vi "FaceRecognition_realtime_detection_usingPCA.vi"() -> ()   [LabVIEW 2017]
uses:
  <vilib>/userdefined/High Color/IMAQdx.ctl
  <vilib>/vision/driver/NI_Vision_Acquisition_Software.lvlib
  <vilib>/vision/NI_Vision_Development_Module.lvlib
panel:
  out "添加的数组":i32[](array[numeric])
  out "Faces":T1[](array[typedef]) {"Rotation" format="%.2f"; "Left" scale=0.0..1024.0; "Right" scale=0.0..1024.0}
  in  "error in":errorcluster
  in  "选项卡控件":enum32{"实时监测", "图像检测"}(tab)
  out "匹配到DB中图像":T2(plugin-control)
  in  "识别方法":u16(ring)=1 items=["模板匹配", "KL变换（调用Matlab）"]
  out "识别结果":string
  in  "是否去背景":bool
  out "Segment image":T2(plugin-control)
  out "检测到人脸":bool
  out "识别时间ms":dbl format="%#.2g"
  in  "切换":bool
  out "Live Image":T2(plugin-control)
  in  "选择相机":T3="cam0"
  in  "停止":bool
  out "Image 2":T2(plugin-control)
  out "识别的图像路径":path
  out "取人脸区域":T2(plugin-control)
  out "识别结果（KL变换）":T2(plugin-control)
  out "输入图像识别结果":string
  out "检测出人脸":bool
  out "Process结果":T2(plugin-control)
  out "Selected img":T2(plugin-control)
  in  "选择图像":bool
  in  "切换 2":bool
  in  "停止2":bool
  # "人脸识别系统"
  # "人脸识别系统"
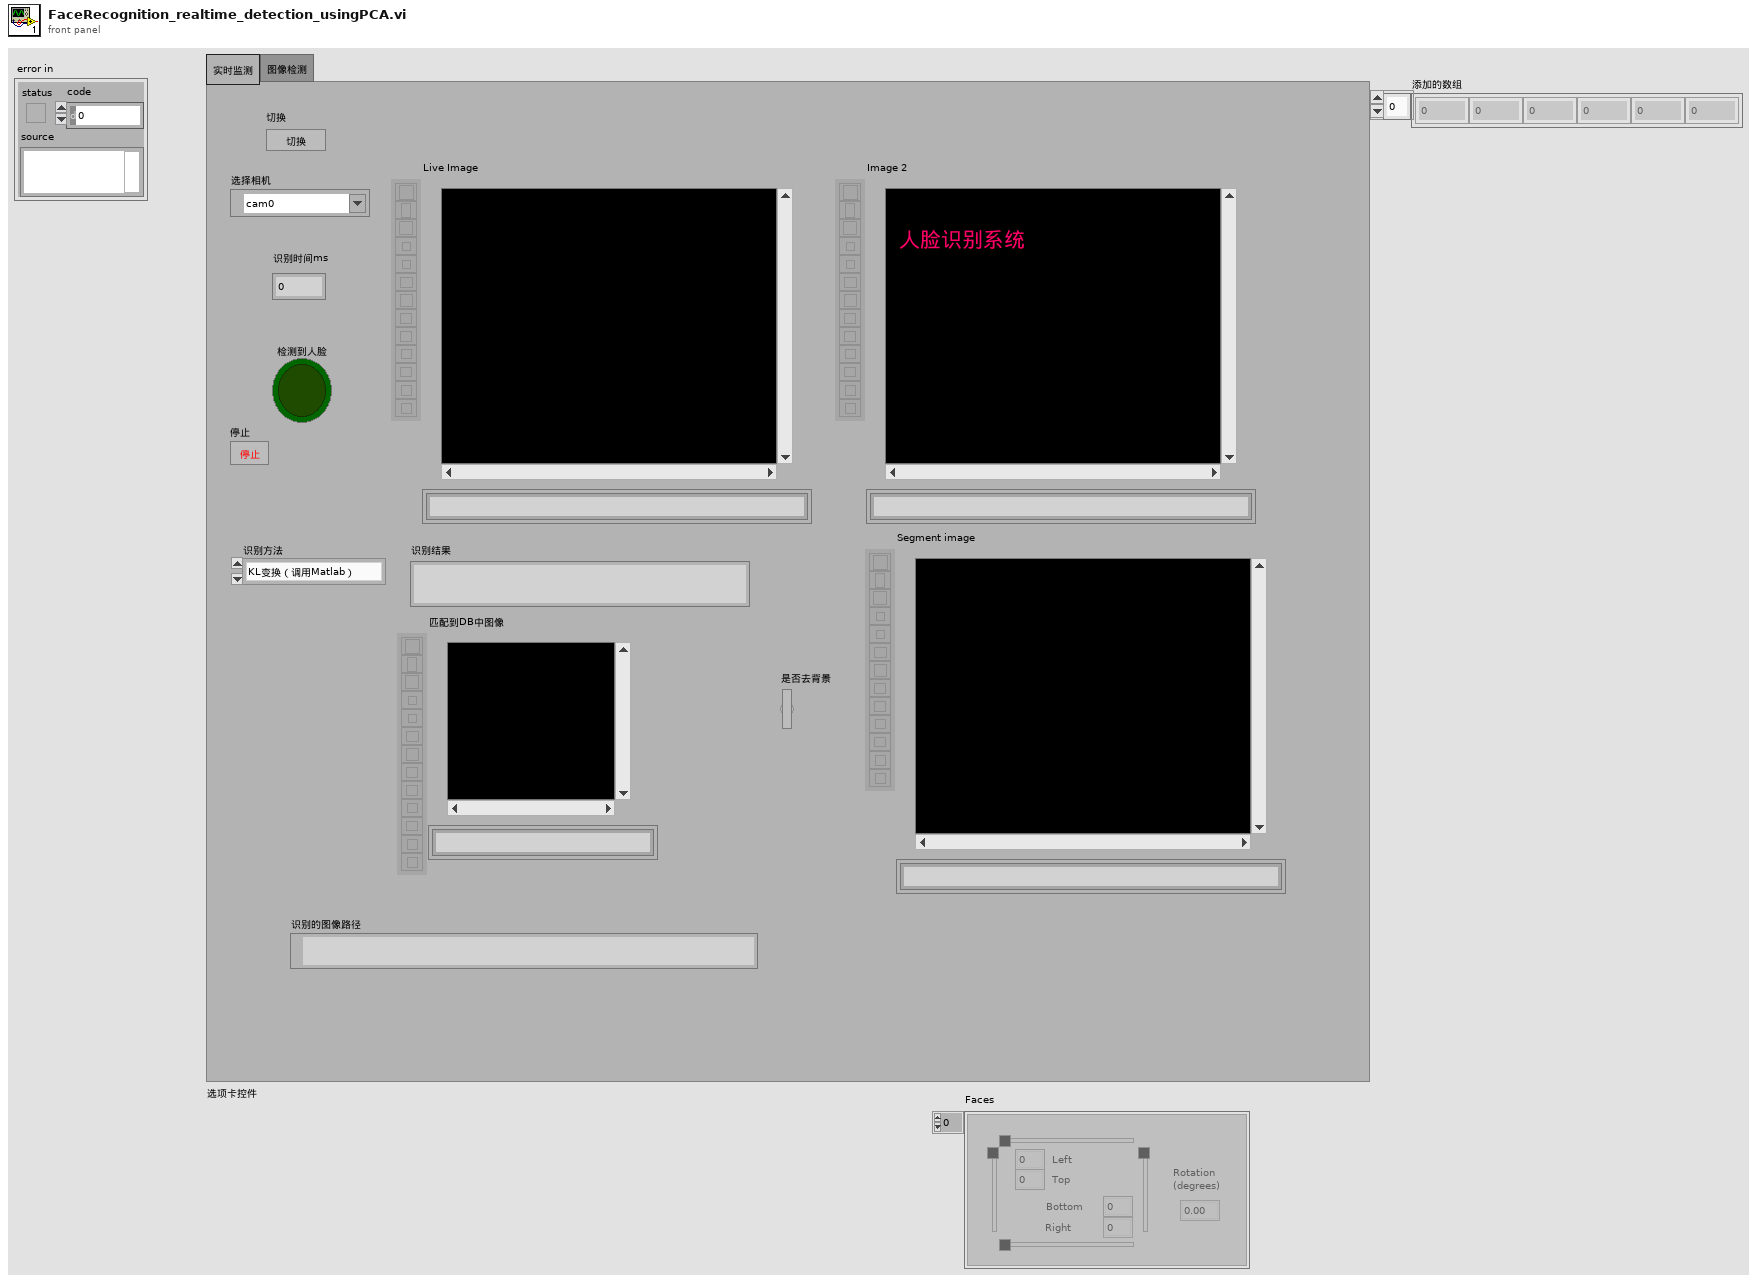
[diagram p1: front panel]
types:
  T1 = typedef "IMAQ Rectangle" = cluster{"Left":i32, "Top":i32, "Right":i32, "Bottom":i32, "Rotation":dbl}
  T2 = typedef "IMAQ Image.ctl" = refnum<image>
  T3 = typedef "IMAQdx.ctl" = refnum<k21>
  T4 = typedef "Image Type" = u32
  T5 = enum32{"Average", "Min", "Max", "Clear  if < ", "Clear  if < or =", "Clear  if =", "Clear  if > or =", "Clear  if >"}
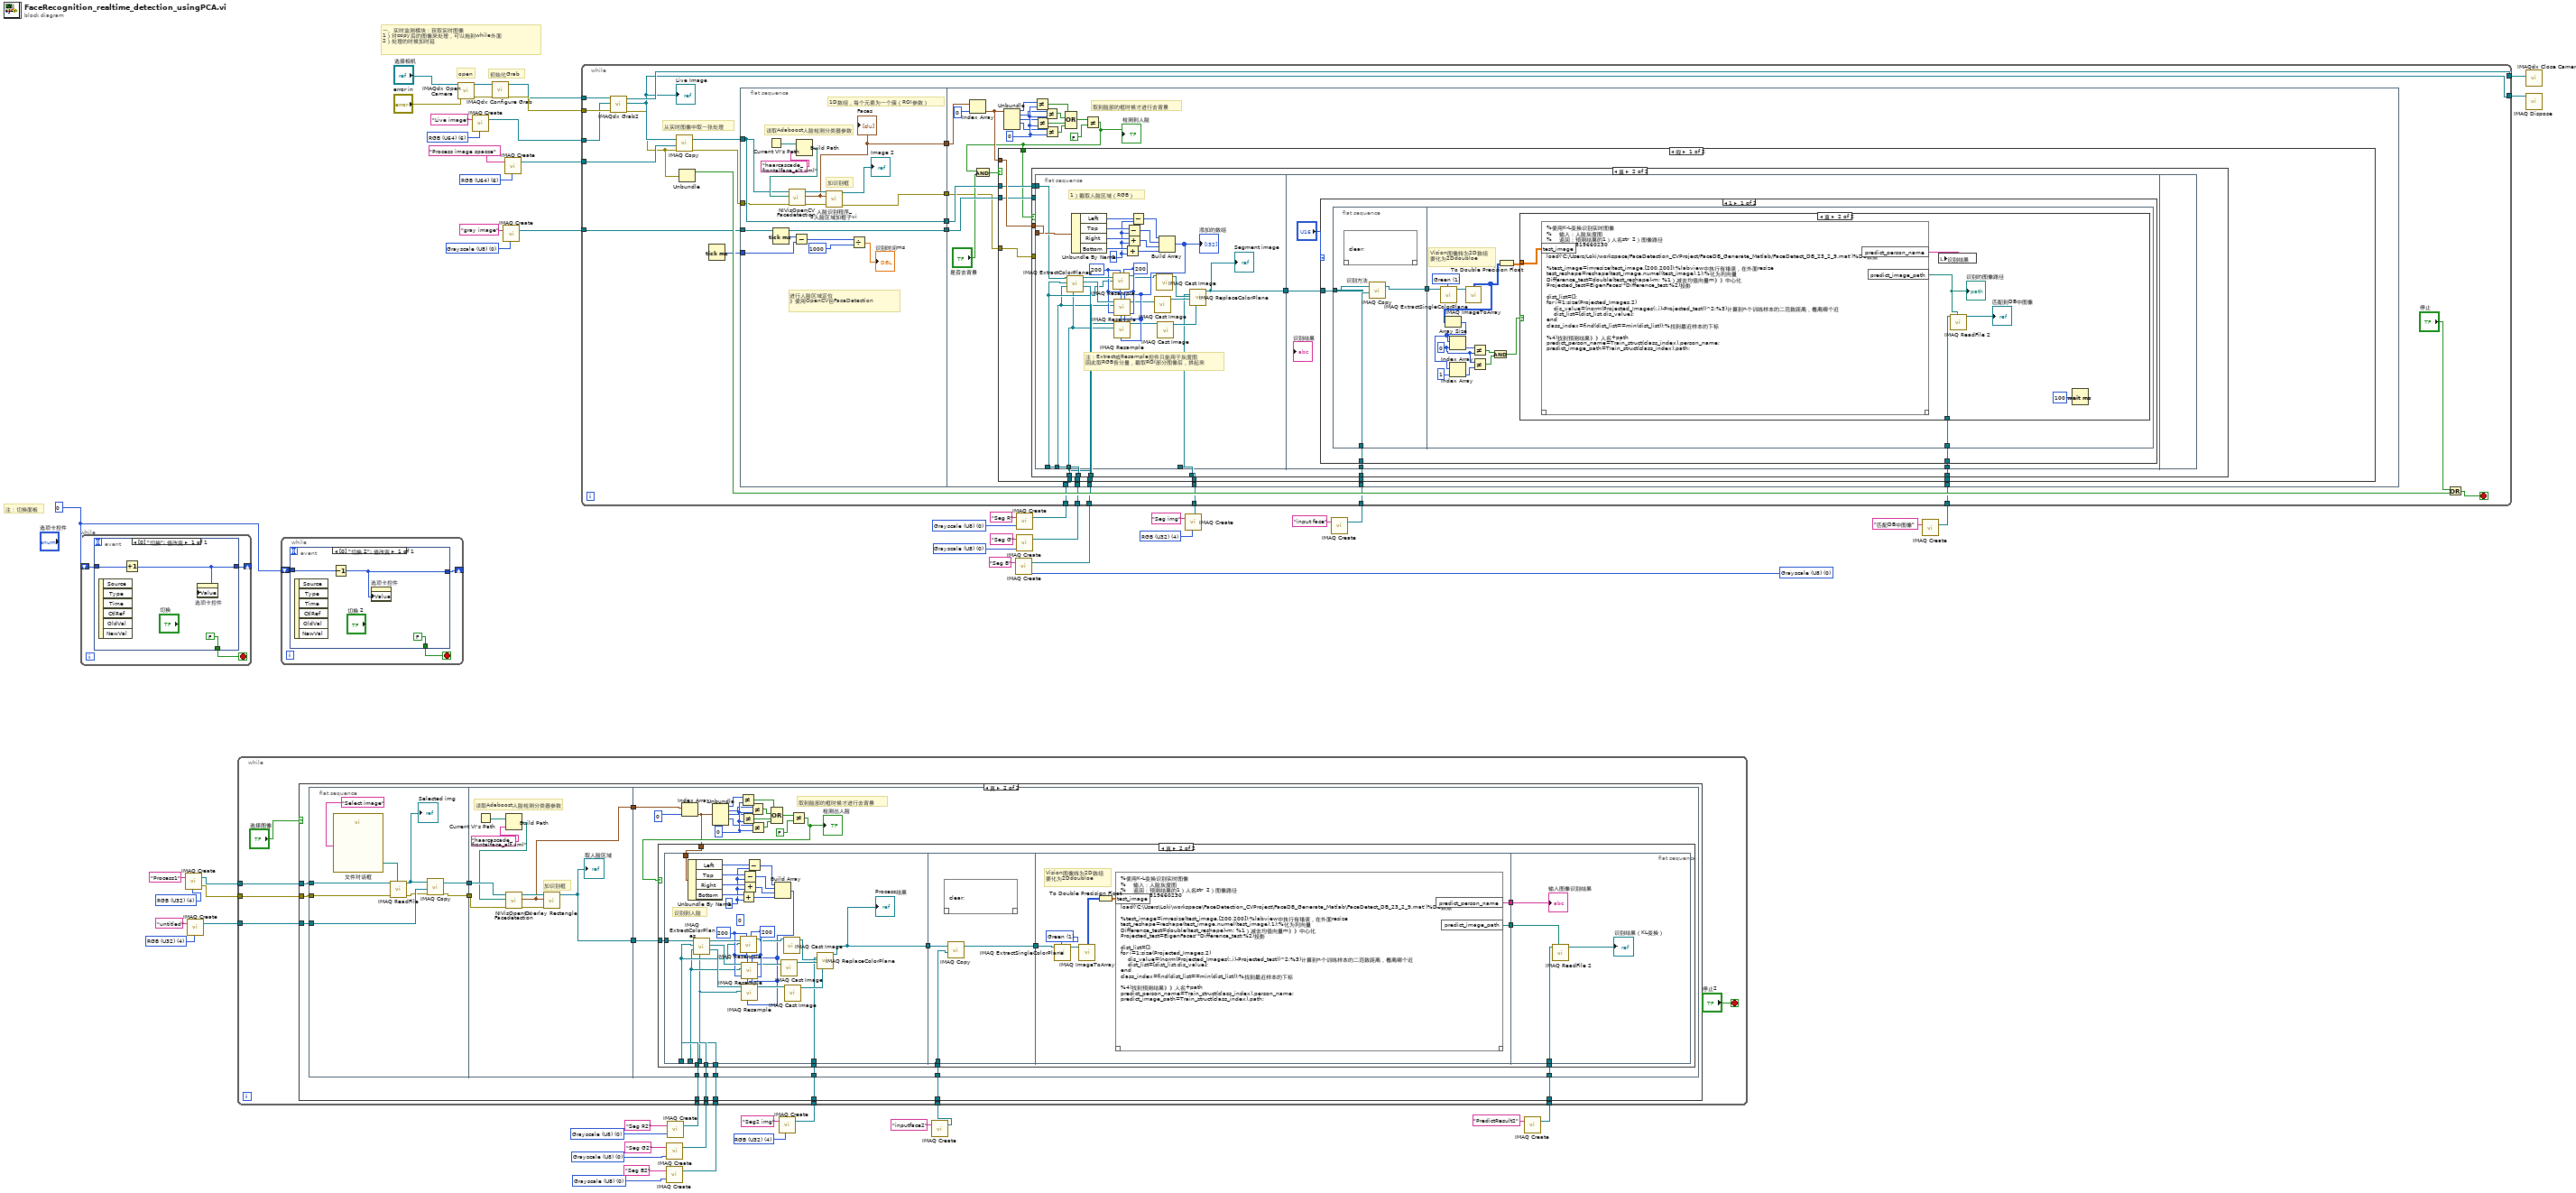
[diagram p0: block diagram]
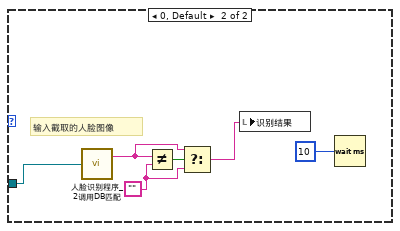
[diagram p6: hidden frame]
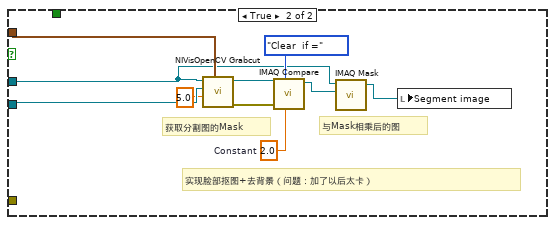
[diagram p7: hidden frame]
diagram:
  w2 = T4 4 items=["Grayscale (U8)", "Grayscale (I16)", "Grayscale (SGL)", "Complex (CSG)", "RGB (U32)", "HSL (U32)", "RGB (U64)", "Grayscale (U16)"] ("Image Type")
  w11 = T4 0 items=["Grayscale (U8)", "Grayscale (I16)", "Grayscale (SGL)", "Complex (CSG)", "RGB (U32)", "HSL (U32)", "RGB (U64)", "Grayscale (U16)"] ("Image Type")
  w12 = T4 0 items=["Grayscale (U8)", "Grayscale (I16)", "Grayscale (SGL)", "Complex (CSG)", "RGB (U32)", "HSL (U32)", "RGB (U64)", "Grayscale (U16)"] ("Image Type")
  w13 = T4 0 items=["Grayscale (U8)", "Grayscale (I16)", "Grayscale (SGL)", "Complex (CSG)", "RGB (U32)", "HSL (U32)", "RGB (U64)", "Grayscale (U16)"] ("Image Type")
  w23 = T4 4 items=["Grayscale (U8)", "Grayscale (I16)", "Grayscale (SGL)", "Complex (CSG)", "RGB (U32)", "HSL (U32)", "RGB (U64)", "Grayscale (U16)"] ("Image Type")
  w28 = T4 0 items=["Grayscale (U8)", "Grayscale (I16)", "Grayscale (SGL)", "Complex (CSG)", "RGB (U32)", "HSL (U32)", "RGB (U64)", "Grayscale (U16)"] ("Image Type")
  w29 = T4 0 items=["Grayscale (U8)", "Grayscale (I16)", "Grayscale (SGL)", "Complex (CSG)", "RGB (U32)", "HSL (U32)", "RGB (U64)", "Grayscale (U16)"] ("Image Type")
  w30 = T4 0 items=["Grayscale (U8)", "Grayscale (I16)", "Grayscale (SGL)", "Complex (CSG)", "RGB (U32)", "HSL (U32)", "RGB (U64)", "Grayscale (U16)"] ("Image Type")
  w35 = T4 0 items=["Grayscale (U8)", "Grayscale (I16)", "Grayscale (SGL)", "Complex (CSG)", "RGB (U32)", "HSL (U32)", "RGB (U64)", "Grayscale (U16)"] ("Image Type")
  w38 = T4 4 items=["Grayscale (U8)", "Grayscale (I16)", "Grayscale (SGL)", "Complex (CSG)", "RGB (U32)", "HSL (U32)", "RGB (U64)", "Grayscale (U16)"] ("Image Type")
  w42 = T4 4 items=["Grayscale (U8)", "Grayscale (I16)", "Grayscale (SGL)", "Complex (CSG)", "RGB (U32)", "HSL (U32)", "RGB (U64)", "Grayscale (U16)"] ("Image Type")
  w44 = 0
  w47 = T4 6 items=["Grayscale (U8)", "Grayscale (I16)", "Grayscale (SGL)", "Complex (CSG)", "RGB (U32)", "HSL (U32)", "RGB (U64)", "Grayscale (U16)"] ("Image Type")
  w45 = T4 6 items=["Grayscale (U8)", "Grayscale (I16)", "Grayscale (SGL)", "Complex (CSG)", "RGB (U32)", "HSL (U32)", "RGB (U64)", "Grayscale (U16)"] ("Image Type")
  # "注：切换面板"
  # "初始化Grab"
  # "open"
  # "一、实时监测模块：获取实时图像\n1）对copy后的图像来处理，可以拖到while外面\n2）处理的时候加时延"
  n1 = while {
    shift-right: [w59] -> _
    shift-left: w44 -> [w60]
    stop <- w58 stop-if-true
    n2 = event shown="[0] \"切换\": 值改变" {
      selector: _ -> [_]
      dyn-events: _ -> [_]
      timeout: _ -> [_]
      tunnel: w60 -> [w63]
      tunnel: [w62] -> w59
      tunnel: [FALSE] -> w58
      event "切换": Value Change {
        n3 = event-data() -> ()  [unwired: 1 in, 6 out]
        n4 = Increment(x=w63) -> (x+1=w62:i32)
        n5 = property on="选项卡控件" class="TabCtl (严格)"("Value"=w62) -> ()  [unwired: 2 in, 2 out]
      }
    }
  }
  n6 = call "IMAQ Create"("Image Name"="Process1", "Image Type"=w42) -> ("New Image"=w41:T2, "error out"=w40:errorcluster)  [unwired: 3 in]
  n7 = call "IMAQ Create"("Image Name"="untitled", "Image Type"=w38) -> ("New Image"=w37:T2)  [unwired: 3 in, 1 out]
  n8 = while {
    shift-right: [w64] -> _
    shift-left: w44 -> [w65]
    stop <- w66 stop-if-true
    n9 = event shown="[0] \"切换 2\": 值改变" {
      selector: _ -> [_]
      dyn-events: _ -> [_]
      timeout: _ -> [_]
      tunnel: [FALSE] -> w66
      tunnel: w65 -> [w68]
      tunnel: [w67] -> w64
      event "切换 2": Value Change {
        n10 = event-data() -> ()  [unwired: 1 in, 6 out]
        n11 = Decrement(x=w68) -> (x-1=w67:i32)
        n12 = property on="选项卡控件" class="TabCtl (严格)"("Value"=w67) -> ()  [unwired: 2 in, 2 out]
      }
    }
  }
  n13 = call <vilib>:"IMAQdx Open Camera.vi"("error in"="error in", "Session In"="选择相机") -> ("error out"=w50:errorcluster, "Session Out"=w49:T3)  [unwired: 8 in]
  n14 = call "IMAQ Create"("Image Name"="Live image", "Image Type"=w45) -> ("New Image"=w54:T2)  [unwired: 3 in, 1 out]
  n15 = call <vilib>:"IMAQdx Configure Grab.vi"("error in"=w50, "Session In"=w49) -> ("error out"=w53:errorcluster, "Session Out"=w52:T3)  [unwired: 8 in]
  n16 = call "IMAQ Create"("Image Name"="gray image", "Image Type"=w35) -> ("New Image"=w34:T2)  [unwired: 3 in, 1 out]
  n17 = call "IMAQ Create"("Image Name"="Process image spacce", "Image Type"=w47) -> ("New Image"=w56:T2)  [unwired: 3 in, 1 out]
  n18 = call "IMAQ Create"("Image Name"="Seg B2", "Image Type"=w11) -> ("New Image"=w8:T2)  [unwired: 3 in, 1 out]
  n19 = call "IMAQ Create"("Image Name"="Seg G2", "Image Type"=w12) -> ("New Image"=w9:T2)  [unwired: 3 in, 1 out]
  n20 = call "IMAQ Create"("Image Name"="Seg R2", "Image Type"=w13) -> ("New Image"=w10:T2)  [unwired: 3 in, 1 out]
  n21 = call "IMAQ Create"("Image Name"="Seg2 img", "Image Type"=w2) -> ("New Image"=w1:T2)  [unwired: 3 in, 1 out]
  n22 = call "IMAQ Create"("Image Name"="inputface2") -> ("New Image"=w6:T2)  [unwired: 4 in, 1 out]
  n23 = call "IMAQ Create"("Image Name"="Seg B", "Image Type"=w28) -> ("New Image"=w25:T2)  [unwired: 3 in, 1 out]
  n24 = call "IMAQ Create"("Image Name"="Seg G", "Image Type"=w29) -> ("New Image"=w26:T2)  [unwired: 3 in, 1 out]
  n25 = call "IMAQ Create"("Image Name"="Seg R", "Image Type"=w30) -> ("New Image"=w27:T2)  [unwired: 3 in, 1 out]
  n26 = call "IMAQ Create"("Image Name"="Seg img", "Image Type"=w23) -> ("New Image"=w22:T2)  [unwired: 3 in, 1 out]
  n27 = call "IMAQ Create"("Image Name"="input face") -> ("New Image"=w20:T2)  [unwired: 4 in, 1 out]
  n28 = call "IMAQ Create"("Image Name"="PredictResult2") -> ("New Image"=w5:T2)  [unwired: 4 in, 1 out]
  n29 = while {
    tunnel: w41 -> [w78]
    tunnel: w40 -> [w77]
    tunnel: w37 -> [w76]
    tunnel: w10 -> [w75]
    tunnel: w9 -> [w74]
    tunnel: w8 -> [w73]
    tunnel: w6 -> [w72]
    tunnel: w5 -> [w71]
    tunnel: w1 -> [w70]
    stop <- "停止2" stop-if-true
    n30 = case shown="真" "选择图像" {
      tunnel: w78 -> [_ w93]
      tunnel: w77 -> [_ w92]
      tunnel: w76 -> [_ w88]
      tunnel: w75 -> [_ w86]
      tunnel: w74 -> [_ w85]
      tunnel: w73 -> [_ w84]
      tunnel: w72 -> [_ w83]
      tunnel: w71 -> [_ w82]
      tunnel: w70 -> [_ w81]
      frame False {
      }
      frame True {
        n31 = flat-sequence {
          tunnel: w93 -> [w101]
          tunnel: w92 -> [w99]
          tunnel: [w96] -> w91
          tunnel: [w94] -> w90
          tunnel: w88 -> [w97]
          tunnel: w91 -> [w110]
          tunnel: w90 -> [w106]
          tunnel: [w104] -> w89
          tunnel: [w103] -> w87
          tunnel: w89 -> [w125]
          tunnel: w87 -> [w118]
          tunnel: w86 -> [w117]
          tunnel: w85 -> [w116]
          tunnel: w84 -> [w115]
          tunnel: w83 -> [w114]
          tunnel: w82 -> [w113]
          tunnel: w81 -> [w112]
          frame #0 {
            n32 = call "文件对话框"("prompt"="Select image") -> ("selected path"=w100:path)  [unwired: 11 in, 3 out]
            n33 = call "IMAQ ReadFile"("File Path"=w100, "error in (no error)"=w99, "Image"=w101) -> ("error out"=w95:errorcluster, "Image Out"=w98:T2)  [unwired: 4 in, 3 out]
            "Selected img" <- w98
            n34 = call "IMAQ Copy"("error in (no error)"=w95, "Image Dst"=w97, "Image Src"=w98) -> ("error out"=w94:errorcluster, "Image Dst Out"=w96:T2)  [unwired: 3 in]
          }
          frame #1 {
            # "加识别框"
            # "读取Adaboost人脸检测分类器参数"
            n35 = Current VI's Path() -> (path=w109:path)
            n36 = Build Path(base path=w109, name or relative path="haarcascade_frontalface_alt.xml") -> (appended path=w107:path)
            n37 = call <vilib>:"NIVisOpenCV Facedetection.vi"("error in (no error)"=w106, "Face Cascade Path"=w107, "Image Src"=w110) -> ("error out"=w105:errorcluster, "Faces"=w104:T1[], "Image Dst Out"=w111:T2)  [unwired: 5 in, 1 out]
            n38 = call "Overlay Rectangle.vi"("error in (no error)"=w105, "Faces"=w104, "Image in"=w111) -> ("Image out"=w103:T2)  [unwired: 7 in, 1 out]
            "取人脸区域" <- w103
          }
          frame #2 {
            w132 = 0 ("y")
            # "取到脸部的框时候才进行去背景"
            n39 = Index Array(array=w125, index=0 ("索引")) -> (element=w119:T1)
            n40 = Unbundle(w119) -> ("Left"=w124:i32, "Top"=w123:i32, "Right"=w121:i32, "Bottom"=w122:i32)  [unwired: 1 out]
            n41 = Not Equal?(x=w124, y=w132) -> (x != y?=w131:bool)
            n42 = Not Equal?(x=w121, y=w132) -> (x != y?=w129:bool)
            n43 = Not Equal?(x=w123, y=w132) -> (x != y?=w130:bool)
            n44 = Not Equal?(x=w122, y=w132) -> (x != y?=w128:bool)
            n45 = Compound Arithmetic op=OR ("复合运算")(w131, w130, w129, w128) -> (w127:bool)
            n46 = Not Equal?(x=w127, y=FALSE) -> (x != y?=w120:bool)
            "检测出人脸" <- w120
            n47 = case shown="真" w120 {
              tunnel: w119 -> [_ w145]
              tunnel: w118 -> [_ w144]
              tunnel: w117 -> [_ w143]
              tunnel: w116 -> [_ w142]
              tunnel: w115 -> [_ w141]
              tunnel: w114 -> [_ w139]
              tunnel: w113 -> [_ w135]
              tunnel: w112 -> [_ w134]
              frame False {
              }
              frame True {
                n48 = flat-sequence {
                  tunnel: w145 -> [w164]
                  tunnel: w144 -> [w152]
                  tunnel: w143 -> [w151]
                  tunnel: w142 -> [w150]
                  tunnel: w141 -> [w149]
                  tunnel: [w148] -> w140
                  tunnel: w134 -> [w147]
                  tunnel: w140 -> [w176]
                  tunnel: w139 -> [w175]
                  tunnel: [w174] -> w138
                  tunnel: w138 -> [w181]
                  tunnel: [w178] -> w137
                  tunnel: [w177] -> w136
                  tunnel: w137 -> [w187]
                  tunnel: w136 -> [w186]
                  tunnel: w135 -> [w185]
                  frame #0 {
                    w159 = 200 ("X Resolution")
                    w160 = 200 ("Y Resolution")
                    (unwired) 0 ("y")
                    w169 = 0 ("y")
                    # "识别到人脸"
                    n49 = Unbundle By Name(w164) -> ("Left"=w173:i32, "Top"=w172:i32, "Right"=w171:i32, "Bottom"=w170:i32)
                    n50 = call "IMAQ ExtractColorPlanes"("Blue or Luma or Val or Inten Plane"=w149, "Green or Sat Plane"=w150, "Red or Hue Plane"=w151, "Image Src"=w152) -> ("Blue or Luma or Val or Inten Plane out"=w161:T2, "Green or Sat Plane out"=w162:T2, "Red or Hue Plane out"=w163:T2)  [unwired: 4 in, 1 out]
                    n51 = Add(x=w170, y=w169) -> (x+y=w165:i32)
                    n52 = Subtract(x=w172, y=w169) -> (x-y=w167:i32)
                    n53 = Add(x=w171, y=w169) -> (x+y=w166:i32)
                    n54 = Subtract(x=w173, y=w169) -> (x-y=w168:i32)
                    n55 = Build Array(w168, w167, w166, w165) -> (w146:i32[])
                    n56 = call "IMAQ Resample"("X Resolution"=w159, "Optional Rectangle"=w146, "Y Resolution"=w160, "Image Dst"=w151, "Image Src"=w163) -> ("Image Dst Out"=w158:T2)  [unwired: 5 in, 1 out]
                    n57 = call "IMAQ Resample"("X Resolution"=w159, "Optional Rectangle"=w146, "Y Resolution"=w160, "Image Dst"=w150, "Image Src"=w162) -> ("Image Dst Out"=w157:T2)  [unwired: 5 in, 1 out]
                    n58 = call "IMAQ Resample"("X Resolution"=w159, "Optional Rectangle"=w146, "Y Resolution"=w160, "Image Dst"=w149, "Image Src"=w161) -> ("Image Dst Out"=w156:T2)  [unwired: 5 in, 1 out]
                    n59 = call "IMAQ Cast Image"("Image Src"=w157) -> ("Image Dst Out"=w153:T2)  [unwired: 9 in, 1 out]
                    n60 = call "IMAQ Cast Image"("Image Src"=w158) -> ("Image Dst Out"=w154:T2)  [unwired: 9 in, 1 out]
                    n61 = call "IMAQ Cast Image"("Image Src"=w156) -> ("Image Dst Out"=w155:T2)  [unwired: 9 in, 1 out]
                    n62 = call "IMAQ ReplaceColorPlane"("Image Dst"=w147, "Red or Hue Plane"=w154, "Green or Sat Plane"=w153, "Blue or Luma or Val or Inten Plane"=w155) -> ("Image Dst Out"=w148:T2)  [unwired: 10 in, 1 out]
                    "Process结果" <- w148
                  }
                  frame #1 {
                    n63 = script code="clear;"() -> ()  [unwired: 1 in, 1 out]
                    n64 = call "IMAQ Copy"("Image Dst"=w175, "Image Src"=w176) -> ("Image Dst Out"=w174:T2)  [unwired: 4 in, 1 out]
                  }
                  frame #2 {
                    w182 = 1 items=["Red", "Green", "Blue", "Hue", "Saturation", "Luminance", "Value", "Intensity"] ("Color Plane")
                    # "Vision图像转为2D数组\n要化为2Ddoubloe"
                    n65 = call "IMAQ ExtractSingleColorPlane"("Color Plane"=w182, "Image Src"=w181) -> ("Image Dst Out"=w183:T2)  [unwired: 8 in, 1 out]
                    n66 = call "IMAQ ImageToArray"("Image"=w183) -> ("Image Pixels (U8)"=w179:u8[][])  [unwired: 3 in, 4 out]
                    n67 = To Double Precision Float(number=w179) -> (double precision float=w180:dbl[][])
                    n68 = script code="%使用K-L变换识别实时图像\n%    输入：人脸灰度图\n%    返回：预测结果的1）人名str  2）图像路径\n% 荀镕基 1819660230\n\nload('C:\\Users\\Loki\\workspace\\FaceDetection_CVProject\\FaceDB_Generate_Matlab\\FaceDetect_DB_23_2_9.mat')%DB数据\n\n%test_image=imresize(test_image,[200,200]);%labview中执行有错误，在外面resize\ntest_reshape=reshape(test_image,numel(test_image),1);%化为列向量\nDifference_test=double(test_reshape)-m; %1）减去均值向量m》》中心化\nProjected_test=EigenFaces'*Difference_test;%2)投影\n\ndist_list=[];\nfor i=1:size(Projected_Images,2)\n    dis_value=(norm(Projected_Images(:,i)-Projected_test))^2;%3)计算到n个训练样本的二范数距离，看离哪个近\n    dist_list=[dist_list,dis_value];\nend\nclass_index=find(dist_list==min(dist_list));%找到最近样本的下标\n\n%4)找到预测结果》》人名+path\npredict_person_name=Train_struct(class_index).person_name;\npredict_image_path=Train_struct(class_index).path;"("test_image"=w180) -> ("predict_person_name"=w178:string, "predict_image_path"=w177:path)  [unwired: 1 in, 1 out]
                  }
                  frame #3 {
                    n69 = call "IMAQ ReadFile 2"("File Path"=w186, "Image"=w185) -> ("Image Out"=→"识别结果（KL变换）":T2)  [unwired: 5 in, 4 out]
                    "输入图像识别结果" <- w187
                  }
                }
              }
            }
          }
        }
      }
    }
  }
  n70 = call "IMAQ Create"("Image Name"="匹配DB中图像") -> ("New Image"=w18:T2)  [unwired: 4 in, 1 out]
  n71 = while {
    tunnel: w52 -> [w211]
    tunnel: w53 -> [w210]
    tunnel: w54 -> [w209]
    tunnel: [w208] -> w55
    tunnel: [w207] -> w21
    tunnel: w56 -> [w206]
    tunnel: w34 -> [w198]
    tunnel: w27 -> [w193]
    tunnel: w26 -> [w192]
    tunnel: w25 -> [w191]
    tunnel: w22 -> [w190]
    tunnel: w20 -> [w189]
    tunnel: w18 -> [w188]
    stop <- w203 stop-if-true
    # "从实时图像中取一张处理"
    n72 = call <vilib>:"IMAQdx Grab2.vi"("error in"=w210, "Image In"=w209, "Session In"=w211) -> ("error out"=w205:errorcluster, "Image Out"=w207:T2, "Session Out"=w208:T3)  [unwired: 5 in, 1 out]
    "Live Image" <- w207
    n73 = call "IMAQ Copy"("error in (no error)"=w205, "Image Dst"=w206, "Image Src"=w207) -> ("error out"=w197:errorcluster, "Image Dst Out"=w201:T2)  [unwired: 3 in]
    n74 = Unbundle(w205) -> ("status"=w204:bool)  [unwired: 2 out]
    n75 = Tick Count (ms)() -> (millisecond timer value=w194:u32)
    n76 = flat-sequence {
      tunnel: w201 -> [w223]
      tunnel: [w223] -> w200
      tunnel: [w224] -> w199
      tunnel: w198 -> [w224]
      tunnel: w197 -> [w222]
      tunnel: [w213] -> w196
      tunnel: [w212] -> w195
      tunnel: w194 -> [w217]
      tunnel: w200 -> [w240]
      tunnel: w199 -> [w239]
      tunnel: w196 -> [w234]
      tunnel: w195 -> [w253]
      tunnel: w193 -> [w233]
      tunnel: w192 -> [w232]
      tunnel: w191 -> [w231]
      tunnel: w190 -> [w230]
      tunnel: w189 -> [w229]
      tunnel: w188 -> [w228]
      frame #0 {
        # "进行人脸区域定位\n》使用OpenCV包FaceDetection"
        # "1D数组，每个元素为一个簇（ROI参数）"
        # "加识别框"
        # "读取Adaboost人脸检测分类器参数"
        n77 = Current VI's Path() -> (path=w227:path)
        n78 = Tick Count (ms)() -> (millisecond timer value=w219:u32)
        n79 = Subtract(x=w219, y=w217) -> (x-y=w220:u32)
        n80 = Build Path(base path=w227, name or relative path="haarcascade_frontalface_alt.xml") -> (appended path=w225:path)
        n81 = call <vilib>:"NIVisOpenCV Facedetection.vi"("error in (no error)"=w222, "Face Cascade Path"=w225, "Image Src"=w223) -> ("error out"=w215:errorcluster, "Faces"=w212:T1[], "Image Dst Out"=w216:T2)  [unwired: 5 in, 1 out]
        "Faces" <- w212
        n82 = call "人脸识别程序_3人脸区域加框子vi.vi"("error in (no error)"=w215, "Faces"=w212, "Image in"=w216) -> ("error out"=w213:errorcluster, "Image out"=→"Image 2":T2)  [unwired: 7 in]
        n83 = Divide(x=w220, y=1000) -> (x/y=→"识别时间ms":dbl)
      }
      frame #1 {
        w251 = 0 ("y")
        # "取到脸部的框时候才进行去背景"
        n84 = Index Array(array=w253, index=0 ("索引")) -> (element=w238:T1)
        n85 = Unbundle(w238) -> ("Left"=w250:i32, "Top"=w249:i32, "Right"=w248:i32, "Bottom"=w247:i32)  [unwired: 1 out]
        n86 = Not Equal?(x=w250, y=w251) -> (x != y?=w246:bool)
        n87 = Not Equal?(x=w248, y=w251) -> (x != y?=w244:bool)
        n88 = Not Equal?(x=w249, y=w251) -> (x != y?=w245:bool)
        n89 = Not Equal?(x=w247, y=w251) -> (x != y?=w243:bool)
        n90 = Compound Arithmetic op=OR ("复合运算")(w246, w245, w244, w243) -> (w242:bool)
        n91 = Not Equal?(x=w242, y=FALSE) -> (x != y?=w235:bool)
        "检测到人脸" <- w235
        n92 = And(x=w235, y="是否去背景") -> (x .and. y?=w236:bool)
        n93 = case shown="假" w236 {
          tunnel: w240 -> [w262 w340]
          tunnel: w239 -> [w263 w348]
          tunnel: w238 -> [w264 w347]
          tunnel: w235 -> [w261 _]
          tunnel: w234 -> [w260 _]
          tunnel: w233 -> [w259 _]
          tunnel: w232 -> [w258 _]
          tunnel: w231 -> [w257 _]
          tunnel: w230 -> [w256 _]
          tunnel: w229 -> [w255 _]
          tunnel: w228 -> [w254 _]
          frame False {
            n94 = case shown="真" w261 {
              tunnel: w264 -> [_ w273]
              tunnel: w263 -> [_ _]
              tunnel: w262 -> [_ w272]
              tunnel: w260 -> [_ _]
              tunnel: w259 -> [_ w271]
              tunnel: w258 -> [_ w270]
              tunnel: w257 -> [_ w269]
              tunnel: w256 -> [_ w268]
              tunnel: w255 -> [_ w266]
              tunnel: w254 -> [_ w265]
              frame False {
              }
              frame True {
                n95 = flat-sequence {
                  tunnel: w273 -> [w301]
                  tunnel: w272 -> [w281]
                  tunnel: w271 -> [w280]
                  tunnel: w270 -> [w275]
                  tunnel: w269 -> [w279]
                  tunnel: w268 -> [w276]
                  tunnel: [w274] -> w267
                  tunnel: w267 -> [w304]
                  tunnel: w266 -> [w303]
                  tunnel: w265 -> [w302]
                  frame #0 {
                    w287 = 200 ("X Resolution")
                    w288 = 200 ("Y Resolution")
                    w296 = 0 ("y")
                    # "1）截取人脸区域（RGB）"
                    # "注：Extract或Resample控件只能用于灰度图\n因此取RGB各分量，截取ROI部分图像后，拼起来"
                    n96 = call "IMAQ ExtractColorPlanes"("Blue or Luma or Val or Inten Plane"=w279, "Green or Sat Plane"=w275, "Red or Hue Plane"=w280, "Image Src"=w281) -> ("Blue or Luma or Val or Inten Plane out"=w289:T2, "Green or Sat Plane out"=w290:T2, "Red or Hue Plane out"=w291:T2)  [unwired: 4 in, 1 out]
                    n97 = Unbundle By Name(w301) -> ("Left"=w300:i32, "Top"=w299:i32, "Right"=w298:i32, "Bottom"=w297:i32)
                    n98 = Add(x=w297, y=w296) -> (x+y=w292:i32)
                    n99 = Subtract(x=w299, y=w296) -> (x-y=w294:i32)
                    n100 = Add(x=w298, y=w296) -> (x+y=w293:i32)
                    n101 = Subtract(x=w300, y=w296) -> (x-y=w295:i32)
                    n102 = Build Array(w295, w294, w293, w292) -> (w286:i32[])
                    "添加的数组" <- w286
                    n103 = call "IMAQ Resample"("X Resolution"=w287, "Optional Rectangle"=w286, "Y Resolution"=w288, "Image Dst"=w280, "Image Src"=w291) -> ("Image Dst Out"=w285:T2)  [unwired: 5 in, 1 out]
                    n104 = call "IMAQ Resample"("X Resolution"=w287, "Optional Rectangle"=w286, "Y Resolution"=w288, "Image Dst"=w275, "Image Src"=w290) -> ("Image Dst Out"=w284:T2)  [unwired: 5 in, 1 out]
                    n105 = call "IMAQ Resample"("X Resolution"=w287, "Optional Rectangle"=w286, "Y Resolution"=w288, "Image Dst"=w279, "Image Src"=w289) -> ("Image Dst Out"=w283:T2)  [unwired: 5 in, 1 out]
                    n106 = call "IMAQ Cast Image"("Image Src"=w284) -> ("Image Dst Out"=w277:T2)  [unwired: 9 in, 1 out]
                    n107 = call "IMAQ Cast Image"("Image Src"=w285) -> ("Image Dst Out"=w278:T2)  [unwired: 9 in, 1 out]
                    n108 = call "IMAQ Cast Image"("Image Src"=w283) -> ("Image Dst Out"=w282:T2)  [unwired: 9 in, 1 out]
                    n109 = call "IMAQ ReplaceColorPlane"("Image Dst"=w276, "Red or Hue Plane"=w278, "Green or Sat Plane"=w277, "Blue or Luma or Val or Inten Plane"=w282) -> ("Image Dst Out"=w274:T2)  [unwired: 10 in, 1 out]
                    "Segment image" <- w274
                  }
                  frame #1 {
                    n110 = case shown="1" "识别方法" {
                      tunnel: w304 -> [w309 w334]
                      tunnel: w303 -> [w307 _]
                      tunnel: w302 -> [w306 _]
                      frame 1 {
                        n111 = flat-sequence {
                          tunnel: w309 -> [w312]
                          tunnel: [w311] -> w308
                          tunnel: w307 -> [w310]
                          tunnel: w308 -> [w314]
                          tunnel: w306 -> [w313]
                          frame #0 {
                            n112 = script code="clear;"() -> ()  [unwired: 1 in, 1 out]
                            n113 = call "IMAQ Copy"("Image Dst"=w310, "Image Src"=w312) -> ("Image Dst Out"=w311:T2)  [unwired: 4 in, 1 out]
                          }
                          frame #1 {
                            w321 = 0 ("索引")
                            w326 = 1 items=["Red", "Green", "Blue", "Hue", "Saturation", "Luminance", "Value", "Intensity"] ("Color Plane")
                            # "Vision图像转为2D数组\n要化为2Ddoubloe"
                            n114 = call "IMAQ ExtractSingleColorPlane"("Color Plane"=w326, "Image Src"=w314) -> ("Image Dst Out"=w325:T2)  [unwired: 8 in, 1 out]
                            n115 = call "IMAQ ImageToArray"("Image"=w325) -> ("Image Pixels (U8)"=w315:u8[][])  [unwired: 3 in, 4 out]
                            n116 = Array Size(array=w315) -> (size(s)=w323:i32[])
                            n117 = Index Array(array=w323, index=w321) -> (element=w322:i32)
                            n118 = Index Array(array=w323, index=1 ("索引")) -> (element=w320:i32)
                            n119 = Not Equal?(x=w322, y=w321) -> (x != y?=w319:bool)
                            n120 = Not Equal?(x=w321, y=w320) -> (x != y?=w318:bool)
                            n121 = And(x=w319, y=w318) -> (x .and. y?=w317:bool)
                            n122 = To Double Precision Float(number=w315) -> (double precision float=w316:dbl[][])
                            n123 = case shown="真" w317 {
                              tunnel: w316 -> [_ w331]
                              tunnel: w313 -> [_ w328]
                              frame False {
                              }
                              frame True {
                                n124 = script code="%使用K-L变换识别实时图像\n%    输入：人脸灰度图\n%    返回：预测结果的1）人名str  2）图像路径\n% 荀镕基 1819660230\n\nload('C:/Users/Loki/workspace/FaceDetection_CVProject/FaceDB_Generate_Matlab/FaceDetect_DB_23_2_9.mat')%DB数据\n\n%test_image=imresize(test_image,[200,200]);%labview中执行有错误，在外面resize\ntest_reshape=reshape(test_image,numel(test_image),1);%化为列向量\nDifference_test=double(test_reshape)-m; %1）减去均值向量m》》中心化\nProjected_test=EigenFaces'*Difference_test;%2)投影\n\ndist_list=[];\nfor i=1:size(Projected_Images,2)\n    dis_value=(norm(Projected_Images(:,i)-Projected_test))^2;%3)计算到n个训练样本的二范数距离，看离哪个近\n    dist_list=[dist_list,dis_value];\nend\nclass_index=find(dist_list==min(dist_list));%找到最近样本的下标\n\n%4)找到预测结果》》人名+path\npredict_person_name=Train_struct(class_index).person_name;\npredict_image_path=Train_struct(class_index).path;"("test_image"=w331) -> ("predict_person_name"=w330:string, "predict_image_path"=w329:path)  [unwired: 1 in, 1 out]
                                "识别的图像路径" <- w329
                                n125 = local write "识别结果"(w330) -> ()
                                n126 = call "IMAQ ReadFile 2"("File Path"=w329, "Image"=w328) -> ("Image Out"=→"匹配到DB中图像":T2)  [unwired: 5 in, 4 out]
                                n127 = Wait (ms)(milliseconds to wait=u32 100 ("等待时间（毫秒）")) -> ()  [unwired: 1 out]
                              }
                            }
                          }
                        }
                      }
                      frame 0, Default {
                        w336 = ""
                        # "输入截取的人脸图像"
                        n128 = call "人脸识别程序_2调用DB匹配.vi"("分割后人脸图像"=w334) -> ("识别结果"=w337:string)  [unwired: 1 out]
                        n129 = Not Equal?(x=w337, y=w336) -> (x != y?=w338:bool)
                        n130 = Select(t=w337, s=w338, f=w336) -> (s? t:f=w333:string)
                        n131 = local write "识别结果"(w333) -> ()
                        n132 = Wait (ms)(milliseconds to wait=10) -> ()  [unwired: 1 out]
                      }
                    }
                  }
                  frame #2 {
                  }
                }
              }
            }
          }
          frame True {
            w344 = sgl 2.0  # Constant
            # "获取分割图的Mask"
            # "与Mask相乘后的图"
            # "实现脸部抠图+去背景（问题：加了以后太卡）"
            n133 = call <vilib>:"NIVisOpenCV Grabcut.vi"("Rectangle"=w347, "Iteration"=5.0, "Image Foreground Mask"=w348, "Image Src"=w340) -> ("error out"=w342:errorcluster, "Image Foreground Mask Out"=w343:T2)  [unwired: 6 in]
            n134 = call "IMAQ Compare"("Constant"=w344, "Operator"=T5."Clear  if =", "error in (no error)"=w342, "Image Src A"=w343) -> ("Image Dst Out"=w341:T2)  [unwired: 6 in, 1 out]
            n135 = call "IMAQ Mask"("Image Mask"=w341, "Image Src"=w340) -> ("Image Dst Out"=w339:T2)  [unwired: 3 in, 1 out]
            n136 = local write "Segment image"(w339) -> ()
          }
        }
      }
    }
    n137 = Or(x="停止", y=w204) -> (x .or. y?=w203:bool)
  }
  n138 = call <vilib>:"IMAQdx Close Camera.vi"("Session In"=w55) -> ()  [unwired: 10 in, 1 out]
  n139 = call "IMAQ Dispose"("Image"=w21) -> ()  [unwired: 5 in, 1 out]
